vi "Teleop.vi"(10 "Match Info":T1={"Autonomous Elapsed Seconds"=0.0, "TeleOp Elapsed Seconds"=0.0, "Disabled Elapsed Seconds"=0.0, "Visited Autonomous"=FALSE, "Visited TeleOp"=FALSE, "Visited Disabled"=FALSE, "Autonomous Settings"={"Autonomous Style"=enum."Independent", "VI Refnum"=refnum}}, 11 "Call Context":T2) -> ()   [LabVIEW 2020]
doc: "This VI is called for each enabled TeleOp packet received from the DS. It is typically used to read from joysticks and other inputs and update I/O or setpoints for timed control loops. It should complete and return within 20 milliseconds or risk missing DS packets."
uses:
  <vilib>/Rock Robotics/Network Tables/NT Write Numeric Array.vi
  <vilib>/Rock Robotics/Network Tables/NT Write Boolean Array.vi
  <vilib>/Rock Robotics/WPI/DriverStation/WPI_DriverStationMatch Info.ctl
  <vilib>/Rock Robotics/WPI/DriverStation/WPI_DriverStationDerivedRobotMode.ctl
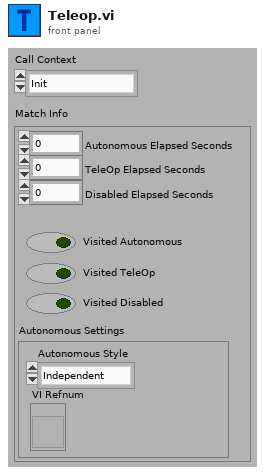
[diagram p1: front panel]
types:
  T1 = typedef "WPI_DriverStationMatch Info.ctl" = cluster{"Autonomous Elapsed Seconds":dbl, "TeleOp Elapsed Seconds":dbl, "Disabled Elapsed Seconds":dbl, "Visited Autonomous":bool, "Visited TeleOp":bool, "Visited Disabled":bool, "Autonomous Settings":cluster{"Autonomous Style":enum16{"Iterative", "Independent"}, "VI Refnum":refnum<vi>}}
  T2 = typedef "WPI_DriverStationDerivedRobotMode.ctl" = enum16{"Init", "Execute", "Stop"}
  T3 = typedef "WPI_JoystickDevRef.ctl" = cluster{"Device":T4}
  T4 = typedef "WPI_JoystickDeviceEnum.ctl" = enum16{"USB 0", "USB 1", "USB 2", "USB 3", "USB 4", "USB 5"}
  T5 = typedef "Command Status Info.ctl" = cluster{"Name":string, "Status":T6, "notifier out":T7}
  T6 = typedef "Completion Status.ctl" = enum16{"Successful", "Aborted", "Incomplete"}
  T7 = typedef "Completion Notifier.ctl" = refnum<notifier>
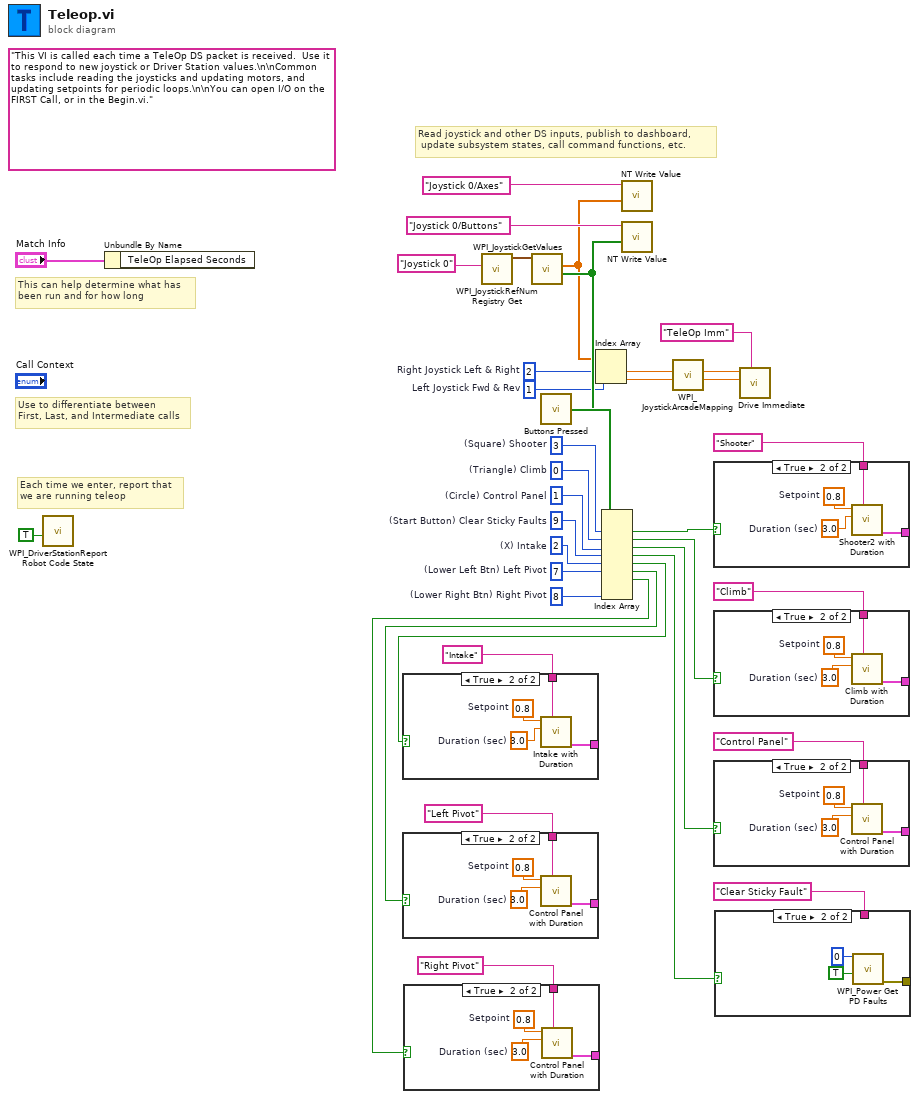
[diagram p0: block diagram]
diagram:
  w1 = 1  # Left Joystick Fwd & Rev
  w2 = 2  # Right Joystick Left & Right
  w3 = 8  # (Lower Right Btn) Right Pivot
  w4 = 7  # (Lower Left Btn) Left Pivot
  w8 = 2  # (X) Intake
  w15 = 9  # (Start Button) Clear Sticky Faults
  w16 = 1  # (Circle) Control Panel
  w17 = 0  # (Triangle) Climb
  w18 = 3  # (Square) Shooter
  (unwired) "This VI is called each time a TeleOp DS packet is received.  Use it to respond to new joystick or Driver Station values.\n\nCommon tasks include reading the joysticks and updating motors, and updating setpoints for periodic loops.\n\nYou can open I/O on the FIRST Call, or in the Begin.vi."
  # "Read joystick and other DS inputs, publish to dashboard,\n update subsystem states, call command functions, etc."
  # "Each time we enter, report that\nwe are running teleop"
  # "Use to differentiate between\nFirst, Last, and Intermediate calls"
  # "This can help determine what has\nbeen run and for how long"
  n1 = call <vilib>:"WPI_DriverStationReport Robot Code State.vi"("TeleOp"=TRUE ("Autonomous")) -> ()  [unwired: 10 in, 1 out]
  n2 = Unbundle By Name("Match Info") -> ()  [unwired: 1 out]
  n3 = call <vilib>:"WPI_JoystickRefNum Registry Get.vi"("refnum name"="Joystick 0") -> ("JoystickDevRef"=w34:T3)  [unwired: 1 in, 9 out]
  n4 = call <vilib>:"WPI_JoystickGetValues.vi"("JoystickDevRef"=w34) -> ("Buttons"=w24:bool[], "Axes"=w23:dbl[])  [unwired: 6 in, 3 out]
  n5 = call "Buttons Pressed.vi"("Button Values"=w24) -> ("Button Presses"=w31:bool[])
  n6 = Index Array(array=w23, index #1=w2, index #2=w1) -> (element #1=w27:dbl, element #2=w26:dbl)
  n7 = Index Array(array=w31, index #1=w18, index #2=w17, index #3=w16, index #4=w15, index #5=w8, index #6=w4, index #7=w3) -> (element #1=w30:bool, element #2=w14:bool, element #3=w13:bool, element #4=w12:bool, element #5=w7:bool, element #6=w6:bool, element #7=w5:bool)  [unwired: 2 in, 2 out]
  n8 = case shown="True" w7 {
    tunnel: "Intake" ("Description") -> [_ w41]
    tunnel: [_ w40] -> _
    frame False {
    }
    frame True {
      w39 = 3.0  # Duration (sec)
      w38 = 0.8  # Setpoint
      n9 = call "Intake with Duration.vi"("Description"=w41, "Duration (s)"=w39, "Setpoint"=w38) -> ("Command Info Out"=w40:T5)  [unwired: 8 in]
    }
  }
  n10 = case shown="True" w6 {
    tunnel: [_ w45] -> _
    tunnel: "Left Pivot" ("Description") -> [_ w44]
    frame False {
    }
    frame True {
      w42 = 3.0  # Duration (sec)
      w43 = 0.8  # Setpoint
      n11 = call "Control Panel with Duration.vi"("Description"=w44, "Duration (s)"=w42, "Setpoint"=w43) -> ("Command Info Out"=w45:T5)  [unwired: 8 in]
    }
  }
  n12 = case shown="True" w5 {
    tunnel: [_ w49] -> _
    tunnel: "Right Pivot" ("Description") -> [_ w48]
    frame False {
    }
    frame True {
      w46 = 3.0  # Duration (sec)
      w47 = 0.8  # Setpoint
      n13 = call "Control Panel with Duration.vi"("Description"=w48, "Duration (s)"=w46, "Setpoint"=w47) -> ("Command Info Out"=w49:T5)  [unwired: 8 in]
    }
  }
  n14 = call-poly <vilib>:"NT Write Value.vi"("Numeric Array"=w23, "Name"="Joystick 0/Axes") -> ()  [unwired: 9 in, 1 out]
  n15 = call-poly <vilib>:"NT Write Value.vi"("Boolean Array"=w24, "Name"="Joystick 0/Buttons") -> ()  [unwired: 9 in, 1 out]
  n16 = call <vilib>:"WPI_JoystickArcadeMapping.vi"("Y axis value"=w26, "X axis value"=w27) -> ("Right Motor Value"=w28:dbl, "Left Motor Value"=w29:dbl)  [unwired: 8 in]
  n17 = case shown="True" w30 {
    tunnel: [_ w53] -> _
    tunnel: "Shooter" ("Description") -> [_ w52]
    frame False {
    }
    frame True {
      w50 = 3.0  # Duration (sec)
      w51 = 0.8  # Setpoint
      n18 = call "Shooter2 with Duration.vi"("Description"=w52, "Duration (s)"=w50, "Setpoint"=w51) -> ("Command Info Out"=w53:T5)  [unwired: 8 in]
    }
  }
  n19 = case shown="True" w14 {
    tunnel: [_ w57] -> _
    tunnel: "Climb" ("Description") -> [_ w56]
    frame False {
    }
    frame True {
      w54 = 3.0  # Duration (sec)
      w55 = 0.8  # Setpoint
      n20 = call "Climb with Duration.vi"("Description"=w56, "Duration (s)"=w54, "Setpoint"=w55) -> ("Command Info Out"=w57:T5)  [unwired: 8 in]
    }
  }
  n21 = case shown="True" w13 {
    tunnel: [_ w61] -> _
    tunnel: "Control Panel" ("Description") -> [_ w60]
    frame False {
    }
    frame True {
      w58 = 3.0  # Duration (sec)
      w59 = 0.8  # Setpoint
      n22 = call "Control Panel with Duration.vi"("Description"=w60, "Duration (s)"=w58, "Setpoint"=w59) -> ("Command Info Out"=w61:T5)  [unwired: 8 in]
    }
  }
  n23 = case shown="True" w12 {
    tunnel: [_ w64] -> _
    tunnel: "Clear Sticky Fault" ("Description") -> [_ _]
    frame False {
    }
    frame True {
      n24 = call <vilib>:"WPI_Power Get PD Faults.vi"("Power Distribution (def)"=u8 0, "Clear Sticky Faults"=TRUE) -> ("error out"=w64:errorcluster)  [unwired: 10 in, 3 out]
    }
  }
  n25 = call "Drive Immediate.vi"("Description"="TeleOp Imm", "Right Setpoint"=w28, "Left Setpoint"=w29) -> ()  [unwired: 8 in, 1 out]
